vi "get_slit_info.vi"(4 "error in (no error)":errorcluster, 6 "mask name":string, 7 "configuration file path":path) -> (0 "error out":errorcluster, 2 "Slit Info":T1 {"Width" format="%.2f"})   [LabVIEW 2015]
uses:
  <vilib>/Utility/config.llb/Read Key (String).vi
  <vilib>/Utility/config.llb/Read Key (Double).vi
  <vilib>/Utility/config.llb/NI_LVConfig.lvlib
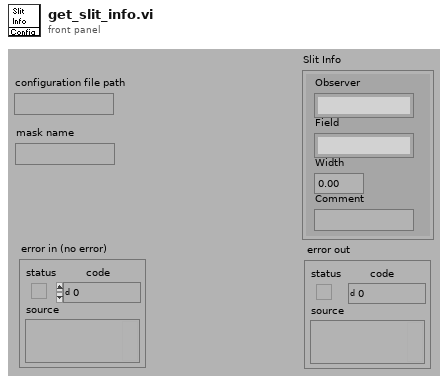
[diagram p1: front panel]
types:
  T1 = cluster{"Comment":string, "Width":dbl, "Observer":string, "Field":string}
  T2 = typedef "NI_LVConfig.lvlib/Config Data RefNum.ctl" = refnum<k1>
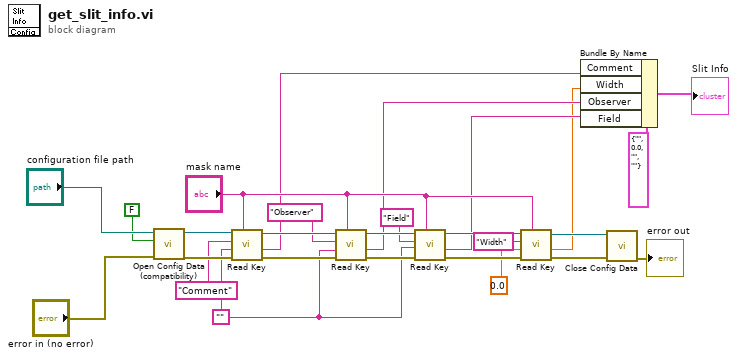
[diagram p0: block diagram]
diagram:
  w8 = ""
  n1 = call <vilib>:"Open Config Data (compatibility).vi"("error in (no error)"="error in (no error)", "create file if necessary (T)"=FALSE, "configuration file path"="configuration file path") -> ("error out"=w27:errorcluster, "refnum"=w26:T2)  [unwired: 6 in, 1 out]
  n2 = call-poly <vilib>:"Read Key.vi"("section"="mask name", "error in (no error)"=w27, "default value"=w8, "key"="Comment", "refnum"=w26) -> ("error out"=w20:errorcluster, "value"=w5:string, "refnum out"=w19:T2)  [unwired: 3 in, 1 out]
  n3 = call-poly <vilib>:"Read Key.vi"("section"="mask name", "error in (no error)"=w20, "default value"=w8, "key"="Observer", "refnum"=w19) -> ("error out"=w16:errorcluster, "value"=w4:string, "refnum out"=w17:T2)  [unwired: 3 in, 1 out]
  n4 = call-poly <vilib>:"Read Key.vi"("section"="mask name", "error in (no error)"=w16, "default value"=w8, "key"="Field", "refnum"=w17) -> ("error out"=w13:errorcluster, "value"=w3:string, "refnum out"=w14:T2)  [unwired: 3 in, 1 out]
  n5 = call-poly <vilib>:"Read Key.vi"("section"="mask name", "error in (no error)"=w13, "default value"=0.0, "key"="Width", "refnum"=w14) -> ("error out"=w10:errorcluster, "value"=w1:dbl, "refnum out"=w9:T2)  [unwired: 3 in, 1 out]
  n6 = Bundle By Name(cluster=T1 {"Comment"="", "Width"=0.0, "Observer"="", "Field"=""} ("Slit Info"), "Comment"=w5, "Width"=w1, "Observer"=w4, "Field"=w3) -> (→"Slit Info":T1)
  n7 = call <vilib>:"Close Config Data.vi"("error in (no error)"=w10, "refnum"=w9) -> ("error out"=→"error out":errorcluster)  [unwired: 8 in, 1 out]
